vi "get_dtype.vi"(11 "String":string) -> (0 "DBL":dbl, 1 "I32":i32, 2 "String out":string, 3 "dtype (0:str, 1:i32, 2:f64)":u32, 4 "IsFloat":bool, 5 "IsNumber":bool)   [LabVIEW 2015, in "oskar_tools.lvlib"]
uses:
  oskar_tools.lvlib
panel:
  out "remaining string":string
  out "error out":errorcluster
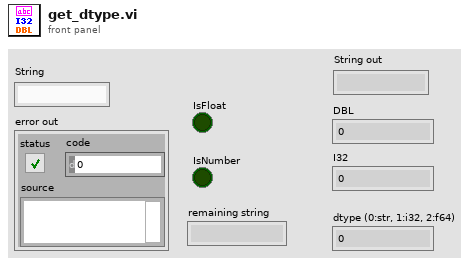
[diagram p1: front panel]
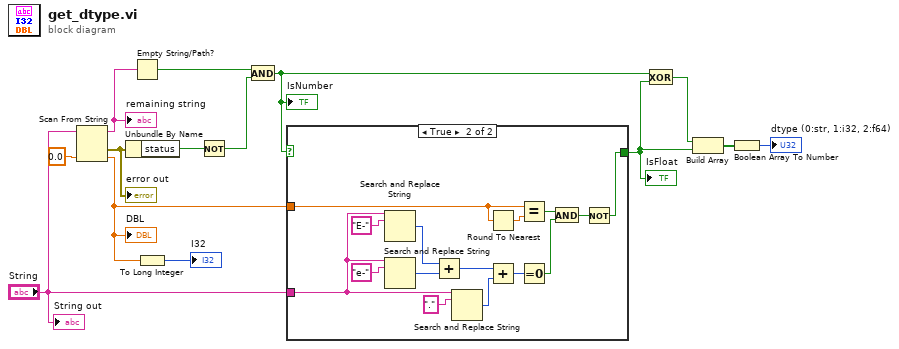
[diagram p0: block diagram]
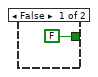
[diagram p2: hidden frame]
diagram:
  n1 = Scan From String(input string="String", default 1=0.0 ("default value 1")) -> (remaining string=w11:string, error out=w13:errorcluster, output 1=w8:dbl)  [unwired: 3 in, 1 out]
  "DBL" <- w8
  "error out" <- w13
  "remaining string" <- w11
  n2 = Unbundle By Name(w13) -> ("status"=w12:bool)
  n3 = Empty String/Path?(string/path=w11) -> (empty?=w10:bool)
  n4 = To Long Integer(number=w8) -> (32bit integer=→"I32":i32)
  n5 = Not(x=w12) -> (.not. x?=w9:bool)
  n6 = And(x=w10, y=w9) -> (x .and. y?=w3:bool)
  "IsNumber" <- w3
  n7 = case shown="True" w3 {
    tunnel: "String" -> [_ w27]
    tunnel: w8 -> [_ w19]
    tunnel: [FALSE w16] -> w2
    frame False {
    }
    frame True {
      n8 = Search and Replace String(input string=w27, search string="E-") -> (number of replacements=w26:i32)  [unwired: 6 in, 3 out]
      n9 = Search and Replace String(input string=w27, search string="e-") -> (number of replacements=w25:i32)  [unwired: 6 in, 3 out]
      n10 = Add(x=w26, y=w25) -> (x+y=w24:i32)
      n11 = Search and Replace String(input string=w27, search string=".") -> (number of replacements=w23:i32)  [unwired: 6 in, 3 out]
      n12 = Round To Nearest(number=w19) -> (nearest integer value=w18:dbl)
      n13 = Add(x=w24, y=w23) -> (x+y=w22:i32)
      n14 = Equal?(x=w19, y=w18) -> (x = y?=w21:bool)
      n15 = Equal To 0?(x=w22) -> (x = 0?=w20:bool)
      n16 = And(x=w21, y=w20) -> (x .and. y?=w17:bool)
      n17 = Not(x=w17) -> (.not. x?=w16:bool)
    }
  }
  "IsFloat" <- w2
  n18 = Exclusive Or(1:w2, 2:w3) -> (0:w1:bool)
  n19 = Build Array(w1, w2) -> (w6:bool[])
  n20 = Boolean Array To Number(Boolean array=w6) -> (number=→"dtype (0:str, 1:i32, 2:f64)":u32)
  "String out" <- "String"
